vi "Write Error Mode.vi"(8 "error in (no error)":errorcluster, 10 "Error Mode":T1, 11 "gScript Interpreter in":refnum<class "gScript Interpreter.lvclass">) -> (0 "error out":errorcluster, 3 "gScript Interpreter out":refnum<class "gScript Interpreter.lvclass">)   [LabVIEW 2023, in "gScript Interpreter.lvclass"]
uses:
  gScript Interpreter.lvclass
  Type Definitions/Error Mode.ctl
  gScript Interpreter.lvclass/gScript Interpreter.ctl
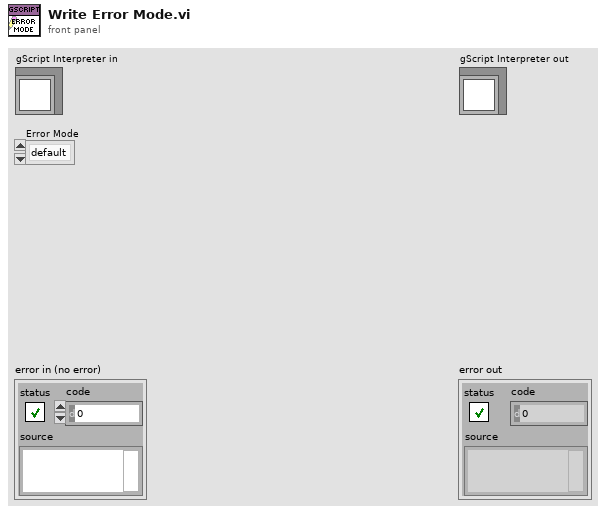
[diagram p1: front panel]
types:
  T1 = typedef "Error Mode.ctl" = enum16{"default", "prompt", "setvar"}
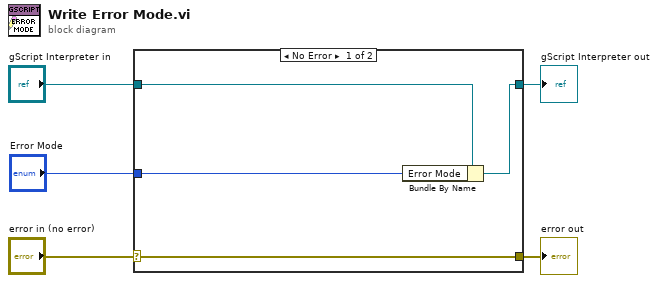
[diagram p0: block diagram]
diagram:
  n1 = case shown="No Error" "error in (no error)" {
    selector: "error in (no error)" -> [w9 w10]
    tunnel: [w9 w10] -> w4
    tunnel: [w7 w11] -> w2
    tunnel: "gScript Interpreter in" -> [w8 w11]
    tunnel: "Error Mode" -> [w6 _]
    frame No Error {
      n2 = Bundle By Name(cluster=w8, "Error Mode"=w6) -> (w7:refnum<class "gScript Interpreter.lvclass">)
    }
    frame Error {
    }
  }
  "error out" <- w4
  "gScript Interpreter out" <- w2
